vi "Apply Wheel State.vi"(8 "error in (no error)":errorcluster, 10 "wheel state in":T1, 11 "wheel in":refnum<class "NI_Robotics_Wheel.lvclass">) -> (0 "error out":errorcluster, 2 "wheel state out":T1, 3 "wheel out":refnum<class "NI_Robotics_Wheel.lvclass">)   [LabVIEW 2017, in "NI_Robotics_Wheel.lvclass"]
uses:
  <vilib>/robotics/Steering/Wheel/NI_Robotics_Wheel.lvclass
  <vilib>/robotics/Steering/Wheel/Wheel State.ctl
  <vilib>/robotics/Steering/Wheel/NI_Robotics_Wheel.lvclass/NI_Robotics_Wheel.ctl
  <vilib>/robotics/Actuation/Motor Communication/Update Motor Velocity Setpoint.vi
  <vilib>/robotics/Actuation/Motor Communication/Check if Valid.vi
  <vilib>/robotics/Utilities/Generate Error.vi
  <vilib>/robotics/Actuation/Motor Communication/NI_Robotics_Motor Communication.lvclass
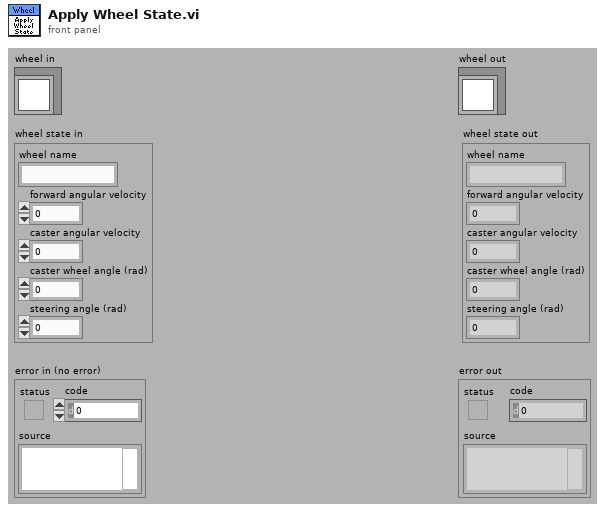
[diagram p1: front panel]
types:
  T1 = typedef "NI_Robotics_Wheel.lvclass/Wheel State.ctl" = cluster{"wheel name":string, "forward angular velocity":dbl, "caster angular velocity":dbl, "caster wheel angle (rad)":dbl, "steering angle (rad)":dbl}
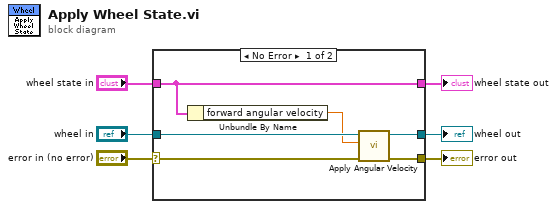
[diagram p0: block diagram]
diagram:
  n1 = case shown="No Error" "error in (no error)" {
    selector: "error in (no error)" -> [w10 w15]
    tunnel: "wheel in" -> [w12 w14]
    tunnel: [w9 w15] -> w1
    tunnel: [w11 w14] -> w5
    tunnel: "wheel state in" -> [w8 w13]
    tunnel: [w8 w13] -> w2
    frame No Error {
      n2 = Unbundle By Name(w8) -> ("forward angular velocity"=w7:dbl)
      n3 = call <vilib>:"Apply Angular Velocity.vi"("error in (no error)"=w10, "forward angular velocity"=w7, "wheel in"=w12) -> ("error out"=w9:errorcluster, "wheel out"=w11:refnum<class "NI_Robotics_Wheel.lvclass">)  [unwired: 7 in]
    }
    frame Error {
    }
  }
  "error out" <- w1
  "wheel out" <- w5
  "wheel state out" <- w2
